vi "Set_VI_Page_Orientation.vi"(2 "error in":errorcluster, 3 "orientation (unchanged)":T1 items=["Unchanged", "portrait", "landscape"], 4 "VI Refnum":refnum<vi>) -> (0 "error out":errorcluster, 1 "VI Refnum out":refnum<vi>)   [LabVIEW 2020, in "NI_ReportGenerationCore.lvlib"]
uses:
  <vilib>/Utility/NIReport.llb/NI_ReportGenerationCore.lvlib
  <vilib>/printing/EasyPrintingControls.llb/orientation.ctl
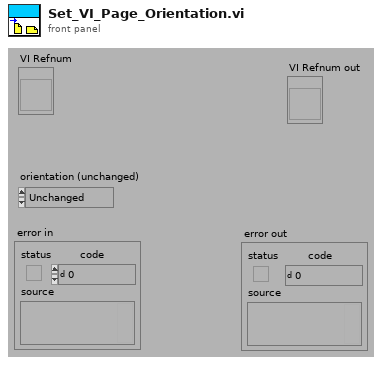
[diagram p1: front panel]
types:
  T1 = typedef "NI_ReportGenerationCore.lvlib/orientation.ctl" = u16
  T2 = enum32{"Portrait", "Landscape", "Rotated Portrait", "Rotated Landscape"}
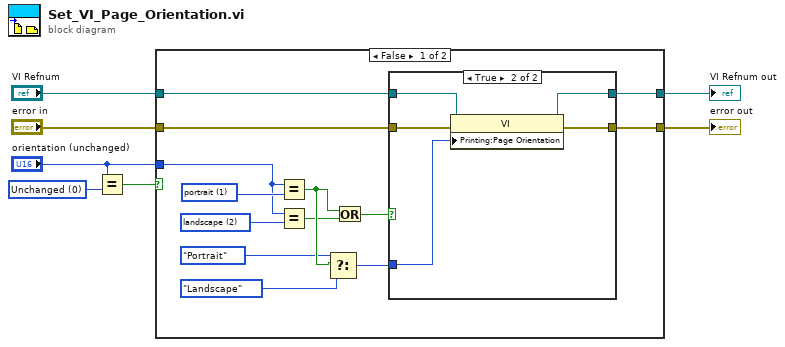
[diagram p0: block diagram]
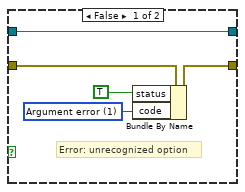
[diagram p2: hidden frame]
diagram:
  w2 = T1 0 items=["Unchanged", "portrait", "landscape"] ("orientation (unchanged)")
  n1 = Equal?(x="orientation (unchanged)", y=w2) -> (x = y?=w4:bool)
  n2 = case shown="False" w4 {
    tunnel: "orientation (unchanged)" -> [w11 _]
    tunnel: "VI Refnum" -> [w15 w32]
    tunnel: "error in" -> [w17 w31]
    tunnel: [w16 w31] -> w7
    tunnel: [w14 w32] -> w3
    frame False {
      w12 = T1 2 items=["Unchanged", "portrait", "landscape"] ("orientation (unchanged)")
      w13 = T1 1 items=["Unchanged", "portrait", "landscape"] ("orientation (unchanged)")
      n3 = Equal?(x=w11, y=w13) -> (x = y?=w20:bool)
      n4 = Equal?(x=w11, y=w12) -> (x = y?=w19:bool)
      n5 = Select(t=T2."Portrait" ("Printing:Page Orientation"), s=w20, f=T2."Landscape" ("Printing:Page Orientation")) -> (s? t:f=w9:T2)
      n6 = Or(x=w20, y=w19) -> (x .or. y?=w18:bool)
      n7 = case shown="True" w18 {
        tunnel: w17 -> [w23 w30]
        tunnel: [w21 w29] -> w16
        tunnel: w15 -> [w22 w27]
        tunnel: [w22 w26] -> w14
        tunnel: w9 -> [_ w28]
        frame False {
          w24 = 1 items=["No error", "Argument error", "Memory is full", "Out of zone", "End of file", "File already open", "Generic file I/O error", "File not found", "File permission error", "Disk is full", "Duplicate path", "Too many files open", "System feature not enabled", "Resource file not found", "Cannot add resource", "Resource not found", "Image not found", "Image memory error", "Pen does not exist", "Config type invalid", "Config token not found", "Config parse error", "Config memory error", "Bad external code format", "Bad external code offset", "External code not present", "Null window", "Destroy window error", "Null menu", "Print aborted", "Bad print record", "Print driver error", "Windows error during printing", "Memory error during printing", "Print dialog error", "Generic print error", "Invalid device refnum", "Device not found", "Device parameter error", "Device unit error", "Cannot open device", "Device call aborted", "Generic error", "Cancelled by user", "Object ID too low", "Object ID too high", "Object not in heap", "Unknown heap", "Unknown object (invalid DefProc)", "Unknown object (DefProc not in table)", "Message out of range", "Invalid (null) method", "Unknown message", "Manager call not supported", "Bad address", "Network operation in progress", "Network operation timed out", "Connection is busy", "Network attribute not supported", "Network error", "Address in use", "System out of memory", "Connection aborted", "Connection refused", "Not connected", "Already connected", "Connection closed", "Initialization error (interapplication manager)", "Bad occurrence", "Wait on unbound occurrence handler", "Occurrence queue overflow", "Datalog type conflict", "Unused", "Unrecognized type (interapplication manager)", "Memory corrupt", "Failed to make temporary DLL", "Old CIN version", "Drag socket not found", "Failed to load drop-object", "Failed to register OLE object", "Failed to release OLE object", "Format specifier type mismatch", "Unknown format specifier", "Too few format specifiers", "Too many format specifiers", "Scan failed", "Newer CIN version", "Error converting to variant", "Runtime menu error", "Password tampered", "Variant attribute not found", "Incompatible variant data type", "Event data is not available", "Event Store is not present", "Occurrence is not found", "Event Queue is not created", "Event info is not available", "Refnum passed is NULL", "Error retrieving Class GUID", "Error retrieving CoClass GUID", "Error retrieving TypeLib GUID.", "Bad built application magic bytes.", "Specific driver is different from the specific driver associated with the Logical Name.", "There is no session opened to the class driver.", "Max Error", "MAX - Error with config objects", "MAX - Error loading configuration", "MAX - Group not supported"]
          # "Error: unrecognized option"
          n8 = Bundle By Name(cluster=w23, "status"=TRUE, "code"=w24) -> (w21:errorcluster)
        }
        frame True {
          n9 = property class="VI"(reference=w27, error in=w30, "Printing:Page Orientation"=w28) -> (reference out=w26:refnum<vi>, error out=w29:errorcluster)
        }
      }
    }
    frame True {
      # "Do not change this setting"
    }
  }
  "VI Refnum out" <- w3
  "error out" <- w7
